vi "1.vi"   [LabVIEW 2023]
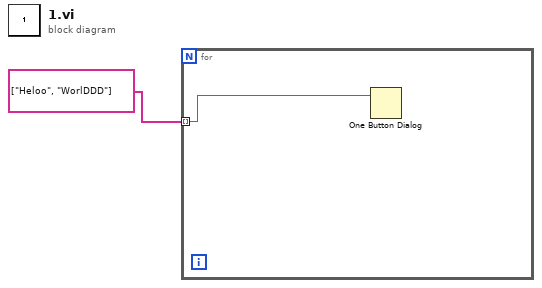
[diagram p0: block diagram]
diagram:
  n1 = for {
    tunnel: string[] ["Heloo", "WorlDDD"] -> [w2] mode=indexing
    n2 = One Button Dialog(message=w2) -> ()  [unwired: 1 in, 1 out]
  }
